vi "WinCI Provider Supports Interface Functionality.vi"(8 "error in (no error)":errorcluster, 10 "interface functionality":T1 items=["REMOVE", "RENAME", "DIFF", "HISTORY", "PROPERTIES", "RUNSCC", "GETCOMMANDOPTIONS", "QUERYINFO", "GETEVENTS", "GETPROJPATH", "ADDFROMSCC", "COMMENTCHECKOUT", "COMMENTCHECKIN", "COMMENTADD", "COMMENTREMOVE", "TEXTOUT", "ADD_STORELATEST", "HISTORY_MULTIFILE", "IGNORECASE", "IGNORESPACE", "POPULATELIST", "COMMENTPROJECT", "DIFFALWAYS", "GET_NOUI", "REENTRANT"]) -> (0 "error out":errorcluster, 2 "provider supports?":bool)   [LabVIEW 2017, in "NI_SCC_WinCI.lvlib"]
uses:
  <vilib>/SourceControl/Providers/WinCI/NI_SCC_WinCI.lvlib
  <vilib>/SourceControl/Providers/WinCI/WinCI Interface Functionality.ctl
  <vilib>/SourceControl/support/SCCSup Message Strings GLBL.vi
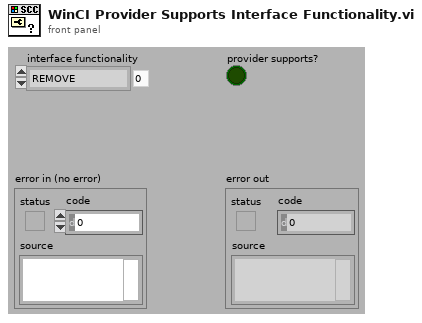
[diagram p1: front panel]
types:
  T1 = typedef "NI_SCC_WinCI.lvlib/WinCI Interface Functionality.ctl" = i32
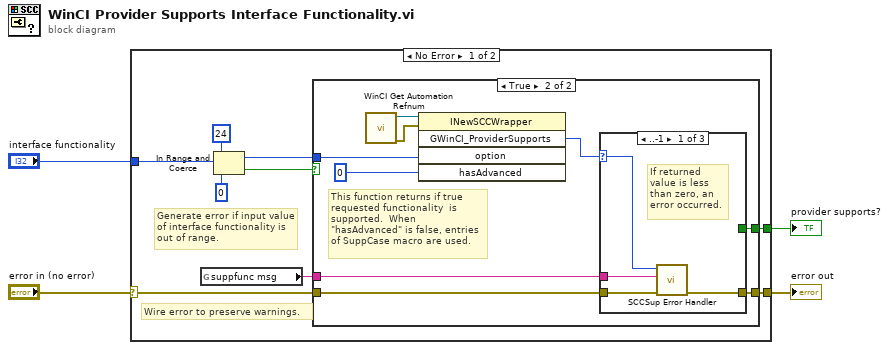
[diagram p0: block diagram]
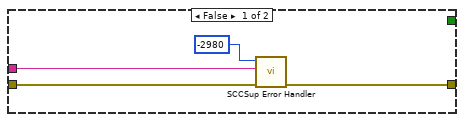
[diagram p2: hidden frame]
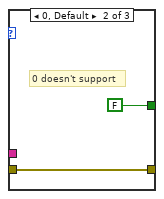
[diagram p3: hidden frame]
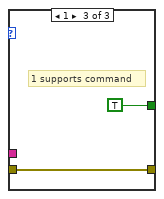
[diagram p4: hidden frame]
diagram:
  n1 = case shown="No Error" "error in (no error)" {
    selector: "error in (no error)" -> [w12 w35]
    tunnel: [w11 w35] -> w3
    tunnel: [w13 _] -> w2
    tunnel: "interface functionality" -> [w7 _]
    frame No Error {
      # "Generate error if input value of interface functionality is out of range."
      # "Wire error to preserve warnings."
      n2 = global read "SCCSup Message Strings GLBL.vi" "suppfunc msg"() -> (w5:string)
      n3 = In Range and Coerce(upper limit=24, x=w7, lower limit=0) -> (coerced(x)=w8:T1, In Range?=w6:bool)
      n4 = case shown="True" w6 {
        tunnel: [_ w26] -> w13
        tunnel: w12 -> [w17 w25]
        tunnel: [w16 w24] -> w11
        tunnel: w8 -> [_ w20]
        tunnel: w5 -> [w15 w23]
        frame False {
          n5 = call <vilib>:"SCCSup Error Handler.vi"("error in (no error)"=w17, "operation message"=w15, "scc error code"=-2980 ("error code")) -> ("error out"=w16:errorcluster)  [unwired: 1 in, 7 out]
        }
        frame True {
          # "This function returns if true requested functionality  is supported.  When \"hasAdvanced\" is false, entries of SuppCase macro are used."
          n6 = call <vilib>:"WinCI Get Automation Refnum.vi"() -> ("error out"=w18:errorcluster, "automation refnum"=w19:refnum<k7>)  [unwired: 10 out]
          n7 = invoke class="INewSCCWrapper" method="GWinCI_ProviderSupports"(reference=w19, error in=w18, "option"=w20, "hasAdvanced"=0) -> ("GWinCI_ProviderSupports"=w22:i32)  [unwired: 1 in, 4 out]
          n8 = case shown="..-1" w22 {
            selector: w22 -> [w28 _ _]
            tunnel: [_ FALSE TRUE] -> w26
            tunnel: w25 -> [w30 w32 w34]
            tunnel: [w29 w32 w34] -> w24
            tunnel: w23 -> [w27 _ _]
            frame ..-1 {
              # "If returned value is less than zero, an error occurred."
              n9 = call <vilib>:"SCCSup Error Handler.vi"("error in (no error)"=w30, "operation message"=w27, "scc error code"=w28) -> ("error out"=w29:errorcluster)  [unwired: 1 in, 7 out]
            }
            frame 0, Default {
              # "0 doesn't support"
            }
            frame 1 {
              # "1 supports command"
            }
          }
        }
      }
    }
    frame Error {
    }
  }
  "error out" <- w3
  "provider supports?" <- w2
